vi "Enqueue Command.vi"(8 "Error In":errorcluster, 10 "Message":string="Open Connection", 11 "Name":string) -> (0 "Error Out":errorcluster)   [LabVIEW 2019, in "Kolmogan Library 1.lvlib"]
uses:
  Kolmogan Library 1.lvlib
  Data Error Notifier/Data and Error Notifier.lvlib
  Queue/Queue.lvlib
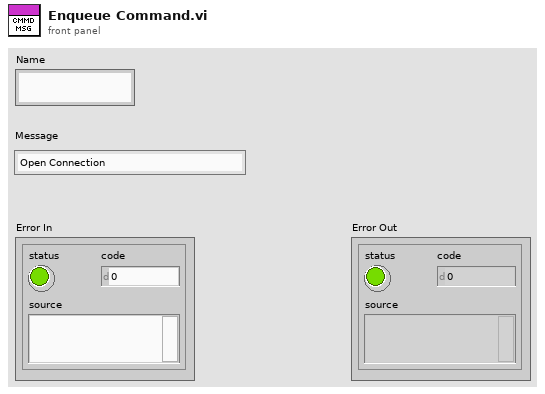
[diagram p1: front panel]
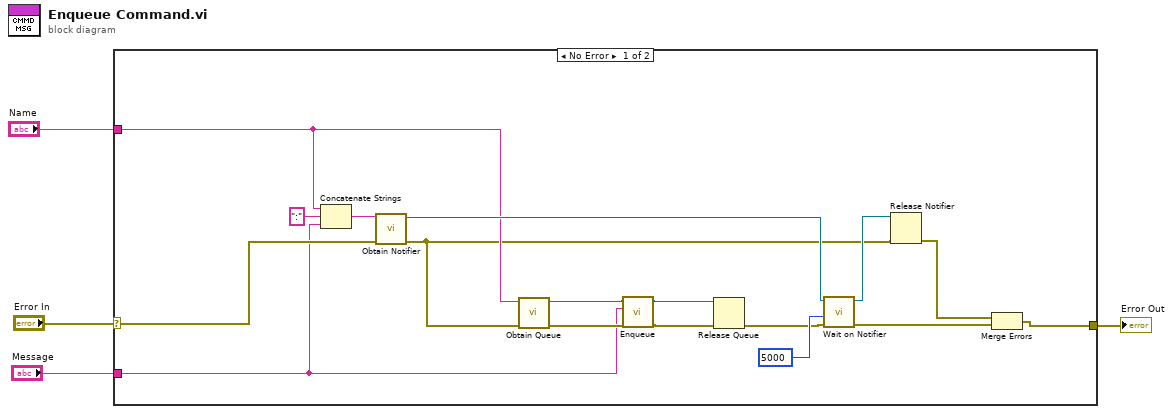
[diagram p0: block diagram]
diagram:
  n1 = case shown="No Error" "Error In" {
    selector: "Error In" -> [w17 w22]
    tunnel: [w19 w22] -> w3
    tunnel: "Name" -> [w11 _]
    tunnel: "Message" -> [w5 _]
    frame No Error {
      n2 = Concatenate Strings(w11, ":" ("string"), w5) -> (w18:string)
      n3 = call "Obtain Notifier.vi"("Error In"=w17, "Name"=w18) -> ("Error Out"=w10:errorcluster, "notifier out"=w12:refnum<notifier>)  [unwired: 8 in]
      n4 = call "Obtain Queue.vi"("Error In"=w10, "Name"=w11) -> ("Error Out"=w6:errorcluster, "queue out"=w9:refnum<queue>)  [unwired: 8 in]
      n5 = call "Enqueue.vi"("Error In"=w6, "Message"=w5, "queue in"=w9) -> ("Error Out"=w8:errorcluster, "queue out"=w7:refnum<queue>)  [unwired: 7 in]
      n6 = Release Queue(queue=w7, error in (no error)=w8) -> (error out=w13:errorcluster)  [unwired: 1 in, 2 out]
      n7 = call "Wait on Notifier.vi"("Error In"=w13, "timeout in ms (-1)"=5000, "notifier in"=w12) -> ("Error Out"=w15:errorcluster, "notifier out"=w16:refnum<notifier>)  [unwired: 6 in, 1 out]
      n8 = Release Notifier(notifier=w16, error in (no error)=w10) -> (error out=w20:errorcluster)  [unwired: 1 in, 2 out]
      n9 = Merge Errors(w20, w15) -> (w19:errorcluster)
    }
    frame Error {
    }
  }
  "Error Out" <- w3
